vi "Kepco cfg reset.vi"(8 "error in (no error)":errorcluster {"code" format="%.0x"}, 9 "Simulation":T1, 10 "Channel parsed command info":T2, 11 "input cluster":refnum<class "KepcoBOP.lvclass">) -> (0 "error out":errorcluster, 2 "new commands":string, 3 "output cluster":refnum<class "KepcoBOP.lvclass">)   [LabVIEW 2013, in "KepcoBOP.lvclass"]
uses:
  KepcoBOP.lvclass
  channel parsed cmd cluster.ctl
  OnOffTypeDef.ctl
  KepcoBOP.lvclass/KepcoBOP.ctl
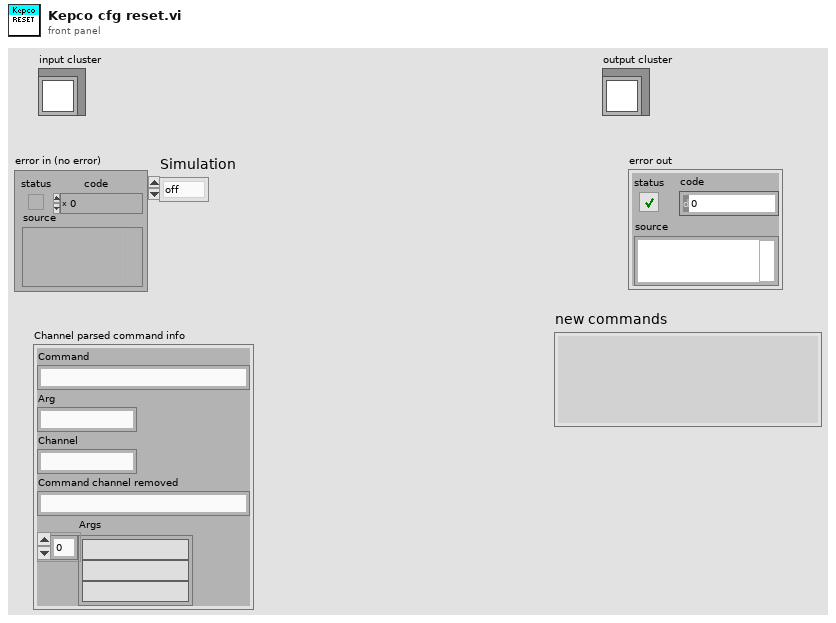
[diagram p1: front panel]
types:
  T1 = typedef "OnOffTypeDef.ctl" = enum16{"off", "on"}
  T2 = typedef "channel parsed cmd cluster.ctl" = cluster{"Command":string, "Arg":string, "Channel":string, "Command channel removed":string, "Args":string[]}
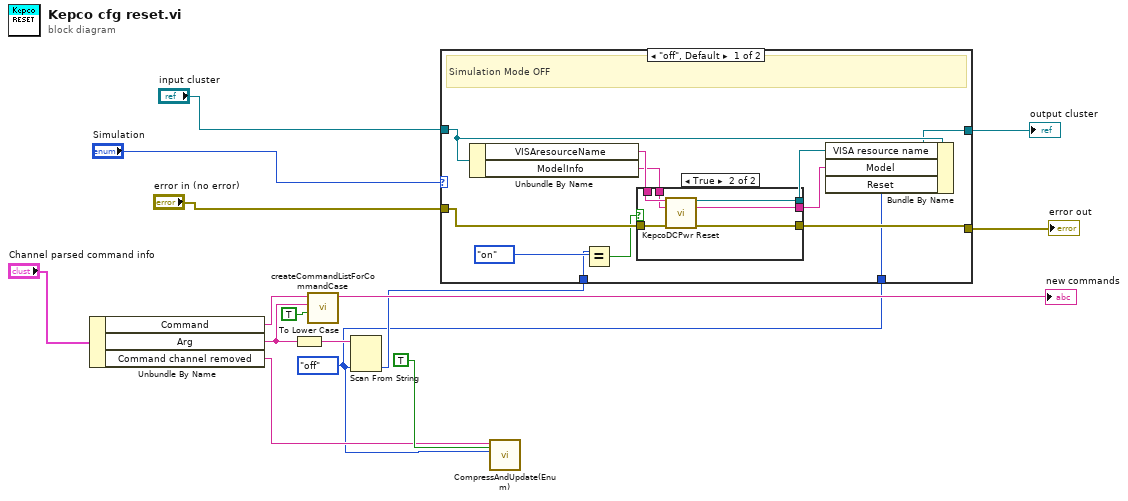
[diagram p0: block diagram]
diagram:
  w1 = enum16{"off", "on"}."off"
  n1 = Unbundle By Name("Channel parsed command info") -> ("Command"=w14:string, "Arg"=w4:string, "Command channel removed"=w2:string)
  n2 = To Lower Case(string=w4) -> (all lower case string=w5:string)
  n3 = call "createCommandListForCommandCase.vi"("immediate Check (only once)"=TRUE, "setvalue"=w4, "command"=w14) -> ("new commands"=→"new commands":string)  [unwired: 8 in]
  n4 = Scan From String(input string=w5, default 1=w1) -> (output 1=w3:enum16{"off", "on"})  [unwired: 3 in, 3 out]
  n5 = case shown="\"off\", Default" "Simulation" {
    tunnel: [w20 w37] -> w9
    tunnel: "input cluster" -> [w27 w38]
    tunnel: "error in (no error)" -> [w21 w37]
    tunnel: [w26 w38] -> w10
    tunnel: w3 -> [w24 _]
    tunnel: w1 -> [w16 _]
    frame "off", Default {
      # "Simulation Mode OFF"
      n6 = Unbundle By Name(w27) -> ("VISAresourceName"=w23:string, "ModelInfo"=w22:string)
      n7 = Equal?(x=w24, y=enum16{"off", "on"}."on") -> (x = y?=w17:bool)
      n8 = case shown="True" w17 {
        tunnel: w23 -> [w29 w36]
        tunnel: w22 -> [w30 w35]
        tunnel: w21 -> [w28 w34]
        tunnel: [w28 w33] -> w20
        tunnel: [w29 w32] -> w19
        tunnel: [w30 w31] -> w18
        frame False {
        }
        frame True {
          n9 = call "KepcoDCPwr Reset.vi"("VISA Session"=w36, "Model In"=w35, "error in (no error)"=w34) -> ("VISA Session Out"=w32:refnum<visa-resource-name>, "Model Out"=w31:string, "error out"=w33:errorcluster)  [unwired: 9 in, 1 out]
        }
      }
      n10 = Bundle By Name(cluster=w27, "VISA resource name"=w19, "Model"=w18, "Reset"=w16) -> (w26:refnum<class "KepcoBOP.lvclass">)
    }
    frame "on" {
      # "Simulation Mode ON"
    }
  }
  "output cluster" <- w10
  "error out" <- w9
  n11 = call "CompressAndUpdate(Enum).vi"("force CVT update (false)"=TRUE ("force CVT update"), "enum variant"=w1, "command or variable name"=w2) -> ()  [unwired: 8 in, 1 out]
